vi "Routing.vi"(4 "Any Data":variant, 6 "Task In":refnum<class "Task Ancestor.lvclass">, 8 "error in (no error)":errorcluster, 9 "Message In":refnum<class "Message.lvclass">, 10 "Actor In":refnum<class "System Actor.lvclass">, 11 "Router in":refnum<class "Router.lvclass">) -> (0 "error out":errorcluster, 2 "Actor Out":refnum<class "System Actor.lvclass">, 3 "Router out":refnum<class "Router.lvclass">)   [LabVIEW 2022 SP3, in "Router.lvclass"]
uses:
  Router.lvclass
  Ancestor Class/Actor/System Actor/System Actor.lvclass
  Ancestor Class/Message/Message.lvclass
  Ancestor Class/Task/Task Ancestor/Task Ancestor.lvclass
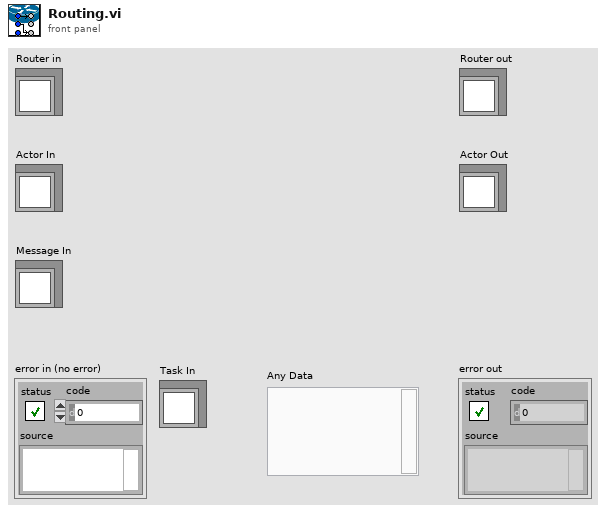
[diagram p1: front panel]
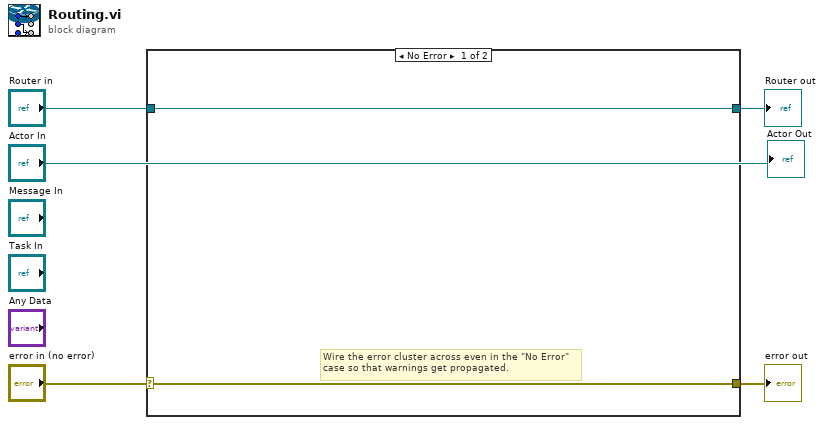
[diagram p0: block diagram]
diagram:
  n1 = case shown="No Error" "error in (no error)" {
    selector: "error in (no error)" -> [w6 w9]
    tunnel: [w6 w9] -> w4
    tunnel: [w7 w8] -> w2
    tunnel: "Router in" -> [w7 w8]
    frame No Error {
      # "Wire the error cluster across even in the \"No Error\"\ncase so that warnings get propagated."
    }
    frame Error {
    }
  }
  "error out" <- w4
  "Router out" <- w2
  "Actor Out" <- "Actor In"
